vi "Write Scheduled.vi"(0 "wait for ack (F)":bool, 1 "scheduled time":timestamp, 5 "element":T1, 7 "element valid? (T)":bool=TRUE, 9 "last element? (F)":bool, 11 "subchannel (0)":i32, 12 "size (unlimited)":i32) -> (3 "actual time":timestamp, 4 "count":i32, 6 "channel":T2, 10 "id":u32)   [LabVIEW 2019, in "MessengerM.lvlib"]
doc: "Writes an element to a Messenger channel at a scheduled time. The endpoint waits until the scheduled time and continues waiting if the channel is full at the scheduled time."
uses:
  MessengerM.lvlib
  ))Channel.ctl
  Element.ctl
  Write With Abort.vi
  Endpoint.vi
  <resource>/ChannelSupport/_ChannelSupport/_ChannelSupport.lvlib
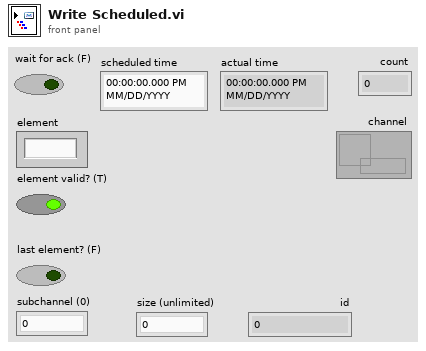
[diagram p1: front panel]
types:
  T1 = typedef "MessengerM.lvlib/Element.ctl" = string
  T2 = typedef "MessengerM.lvlib/))Channel.ctl" = refnum<queue>
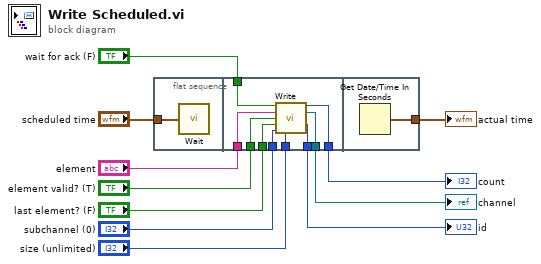
[diagram p0: block diagram]
diagram:
  n1 = flat-sequence {
    tunnel: "scheduled time" -> [w12]
    tunnel: "element" -> [w21]
    tunnel: "size (unlimited)" -> [w18]
    tunnel: [w20] -> w7
    tunnel: [w19] -> w6
    tunnel: "wait for ack (F)" -> [w17]
    tunnel: "subchannel (0)" -> [w16]
    tunnel: "last element? (F)" -> [w15]
    tunnel: [w14] -> w2
    tunnel: "element valid? (T)" -> [w13]
    tunnel: [w22] -> w10
    frame #0 {
      n2 = call <resource>:"Wait.vi"("desired time"=w12) -> ()  [unwired: 2 out]
    }
    frame #1 {
      n3 = call "Write.vi"("wait for ack (F)"=w17, "element"=w21, "element valid? (T)"=w13, "last element? (F)"=w15, "subchannel (0)"=w16, "size (unlimited)"=w18) -> ("count"=w14:i32, "channel"=w20:T2, "id"=w19:u32)  [unwired: 6 in, 1 out]
    }
    frame #2 {
      n4 = Get Date/Time In Seconds() -> (seconds since 1Jan1904=w22:timestamp)
    }
  }
  "channel" <- w7
  "actual time" <- w10
  "id" <- w6
  "count" <- w2
